vi "parse by space_v2019_07_18.vi"(8 "error in (no error)":errorcluster, 11 "String":string) -> (0 "error out":errorcluster, 3 "Array":string[](array[string]))   [LabVIEW 2016]
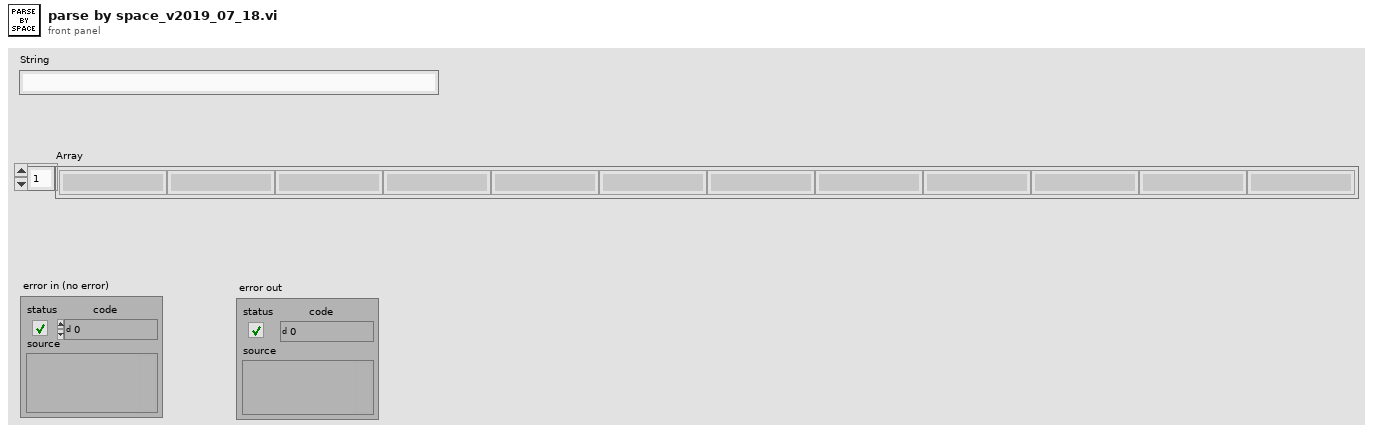
[diagram p1: front panel]
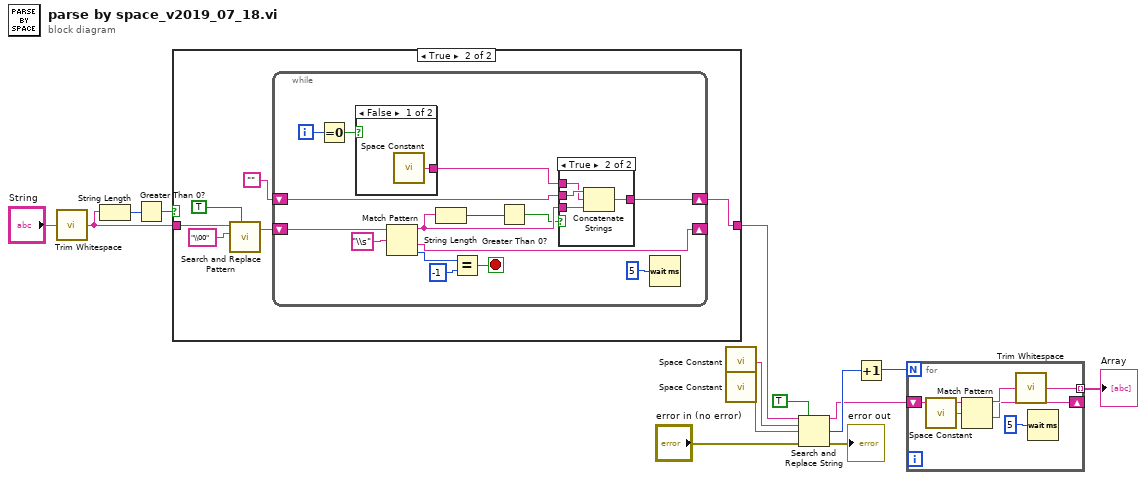
[diagram p0: block diagram]
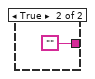
[diagram p3: hidden frame]
diagram:
  n1 = call <vilib>:"Trim Whitespace.vi"("string"="String") -> ("trimmed string"=w1:string)  [unwired: 1 in]
  n2 = String Length(string=w1) -> (length=w2:i32)
  n3 = Greater Than 0?(x=w2) -> (x > 0?=w3:bool)
  n4 = case shown="True" w3 {
    tunnel: [w15 w21] -> w4
    tunnel: w1 -> [w15 w19]
    frame False {
    }
    frame True {
      n5 = call <vilib>:"Search and Replace Pattern.vi"("string"=w19, "regular expression (\"\")"="\\00" ("search string"), "replace all? (F)"=TRUE) -> ("result string"=w17:string)  [unwired: 2 in, 1 out]
      n6 = while {
        shift-right: [w35] -> _
        shift-left: w17 -> [w22]
        shift-right: [w33] -> w21
        shift-left: "" -> [w34]
        i -> [w32]
        stop <- w36 stop-if-true
        n7 = Equal To 0?(x=w32) -> (x = 0?=w25:bool)
        n8 = case shown="False" w25 {
          tunnel: [w37 ""] -> w24
          frame False {
            n9 = call <vilib>:"Space Constant.vi"() -> ("String"=w37:string)
          }
          frame True {
          }
        }
        n10 = Match Pattern(string=w22, regular expression="\\s") -> (before substring=w28:string, after substring=w35:string, offset past match=w30:i32)  [unwired: 1 in, 1 out]
        n11 = String Length(string=w28) -> (length=w27:i32)
        n12 = Equal?(x=w30, y=-1) -> (x = y?=w36:bool)
        n13 = Greater Than 0?(x=w27) -> (x > 0?=w26:bool)
        n14 = case shown="True" w26 {
          tunnel: w34 -> [w39 w43]
          tunnel: w28 -> [_ w42]
          tunnel: [w39 w41] -> w33
          tunnel: w24 -> [_ w40]
          frame False {
          }
          frame True {
            n15 = Concatenate Strings(w43, w40, w42) -> (w41:string)
          }
        }
        n16 = Wait (ms)(milliseconds to wait=u32 5) -> ()  [unwired: 1 out]
      }
    }
  }
  n17 = call <vilib>:"Space Constant.vi"() -> ("String"=w14:string)
  n18 = call <vilib>:"Space Constant.vi"() -> ("String"=w13:string)
  n19 = Search and Replace String(replace all?=TRUE ("ignore case? (F)"), input string=w4, search string=w14, replace string=w13, error in="error in (no error)") -> (result string=w9:string, number of replacements=w11:i32, error out=→"error out":errorcluster)  [unwired: 3 in, 1 out]
  n20 = Increment(x=w11) -> (x+1=w10:i32)
  n21 = for {
    N: w10 -> [_]
    shift-right: [w45] -> _
    shift-left: w9 -> [w49]
    tunnel: [w44] -> w6 mode=indexing
    n22 = call <vilib>:"Space Constant.vi"() -> ("String"=w48:string)
    n23 = Match Pattern(string=w49, regular expression=w48) -> (before substring=w46:string, after substring=w45:string)  [unwired: 1 in, 2 out]
    n24 = call <vilib>:"Trim Whitespace.vi"("string"=w46) -> ("trimmed string"=w44:string)  [unwired: 1 in]
    n25 = Wait (ms)(milliseconds to wait=u32 5) -> ()  [unwired: 1 out]
  }
  "Array" <- w6
